vi "dataValueToXml.vi"(8 "error in (no error)":errorcluster, 11 "ScriptEvent in":refnum<class "ScriptEvent.lvclass">) -> (0 "error out":errorcluster, 2 "dataValueXml":refnum<class "xmlNode.lvclass">, 3 "ScriptEvent out":refnum<class "ScriptEvent.lvclass">)   [LabVIEW 2011, in "Tools.lvlib" / "Scripting.lvlib" / "ScriptEvent.lvclass"]
uses:
  ScriptEvent.lvclass
  xmlNode/xmlNode.lvclass
  ScriptEvent.lvclass/ScriptEvent.ctl
  DatabaseHelpers/Database Objects/Channel/Channel.lvclass
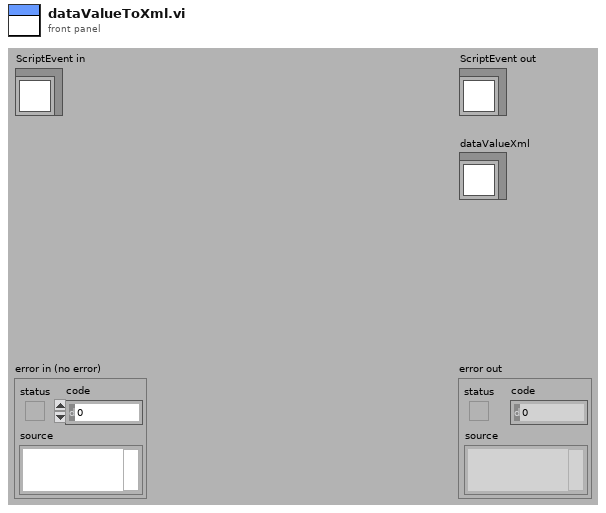
[diagram p1: front panel]
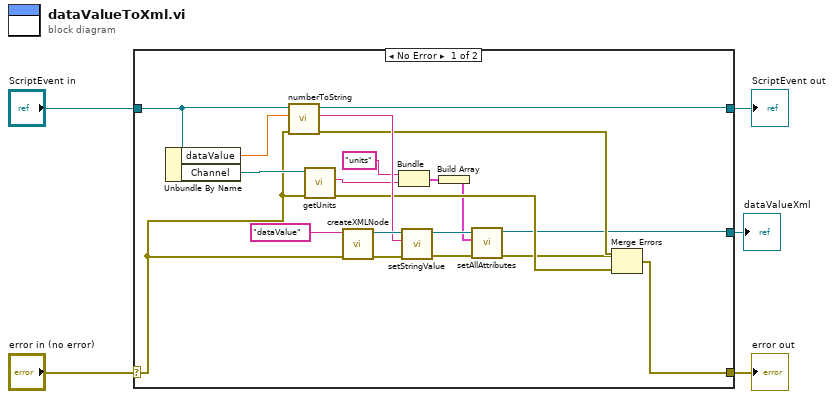
[diagram p0: block diagram]
diagram:
  n1 = case shown="No Error" "error in (no error)" {
    selector: "error in (no error)" -> [w15 w27]
    tunnel: [w17 w27] -> w4
    tunnel: [w19 w26] -> w2
    tunnel: "ScriptEvent in" -> [w20 w26]
    tunnel: [w7 _] -> w1
    frame No Error {
      n2 = Unbundle By Name(w20) -> ("dataValue"=w22:dbl, "Channel"=w16:refnum<class "Channel.lvclass">)
      n3 = call "numberToString.vi"("error in (no error)"=w15, "Numeric"=w22, "ScriptEvent in"=w20) -> ("error out"=w18:errorcluster, "String"=w21:string, "ScriptEvent out"=w19:refnum<class "ScriptEvent.lvclass">)  [unwired: 6 in]
      n4 = call-dynamic "getUnits.vi"("error in (no error)"=w15, "Channel.lvclass in"=w16) -> ("error out"=w14:errorcluster, "units"=w11:string)  [unwired: 7 in, 1 out]
      n5 = call "createXMLNode.vi"("error in (no error)"=w15, "name"="dataValue") -> ("error out"=w23:errorcluster, "xmlNode out"=w24:refnum<class "xmlNode.lvclass">)  [unwired: 8 in]
      n6 = Bundle("units", "units"=w11) -> (w9:cluster{string, "units":string})  [unwired: 1 in]
      n7 = call-dynamic "setStringValue.vi"("error in (no error)"=w23, "stringValue"=w21, "xmlNode.lvclass in"=w24) -> ("error out"=w13:errorcluster, "xmlNode.lvclass out"=w12:refnum<class "xmlNode.lvclass">)  [unwired: 7 in]
      n8 = Build Array(w9) -> (w8:cluster{string, "units":string}[])
      n9 = call-dynamic "setAllAttributes.vi"("error in (no error)"=w13, "attributes"=w8, "xmlNode in"=w12) -> ("error out"=w6:errorcluster, "xmlNode out"=w7:refnum<class "xmlNode.lvclass">)  [unwired: 7 in]
      n10 = Merge Errors(w18, w6, w14) -> (w17:errorcluster)
    }
    frame Error {
    }
  }
  "error out" <- w4
  "ScriptEvent out" <- w2
  "dataValueXml" <- w1
